vi "Init Open Error Logs Folder Button.vi"(8 "Error In":errorcluster, 10 "Error_Log_Setting":T1, 11 "Open Error Logs Folder Button Reference":refnum<vi>) -> (0 "Error Out":errorcluster)   [LabVIEW 2023, in "Error Manager.lvlib"]
doc: "Blank VI with error handling."
uses:
  Error Manager.lvlib
  Settings/Error_Log_Setting (enum).ctl
  Settings/Settings.lvclass
panel:
  # "Input\nInputs to the VI"
  # "Development\nControls or indicators that are useful for development or testing, but which are not outputs of the VI."
  # "Output\nOutputs of the VI"
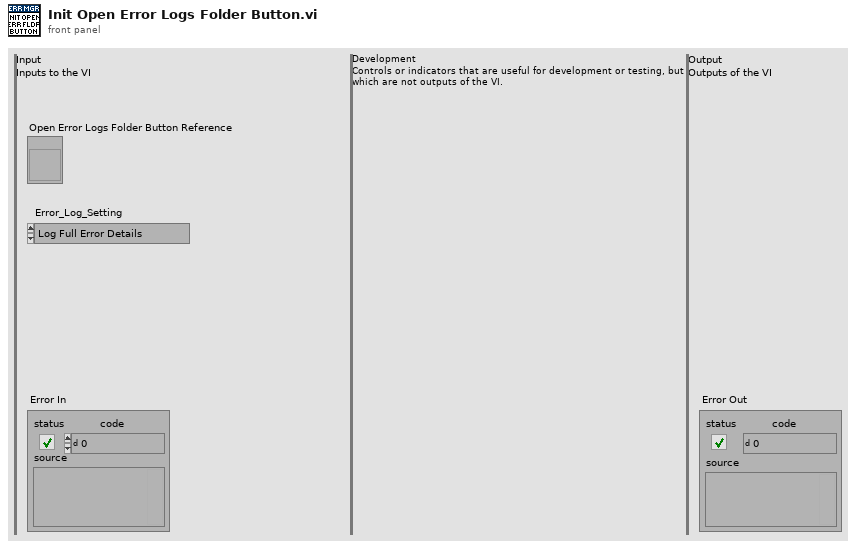
[diagram p1: front panel]
types:
  T1 = typedef "Error Manager.lvlib/Settings.lvclass/Error_Log_Setting (enum).ctl" = enum16{"Log Full Error Details", "Log Error Codes Only", "Do Not Log"}
  T2 = enum8{"Enabled", "Disabled", "Disabled and Grayed Out"}
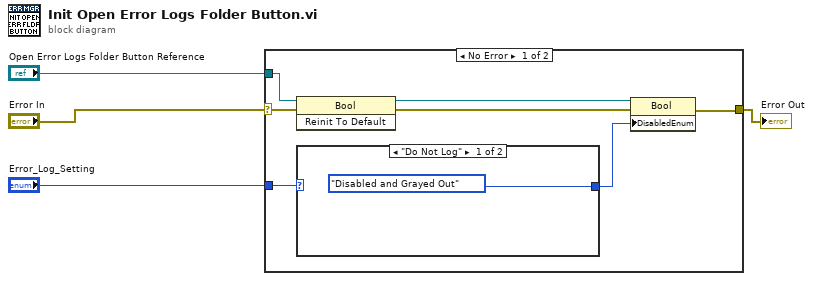
[diagram p0: block diagram]
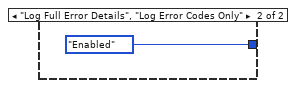
[diagram p2: hidden frame]
diagram:
  n1 = case shown="No Error" "Error In" {
    selector: "Error In" -> [w11 w14]
    tunnel: [w10 w14] -> w3
    tunnel: "Open Error Logs Folder Button Reference" -> [w6 _]
    tunnel: "Error_Log_Setting" -> [w9 _]
    frame No Error {
      n2 = invoke class="Bool" method="Reinit To Default"(reference=w6, error in=w11) -> (reference out=w5:refnum<vi>, error out=w7:errorcluster)  [unwired: 1 in, 1 out]
      n3 = case shown="\"Do Not Log\"" w9 {
        tunnel: [T2."Disabled and Grayed Out" ("Disabled") T2."Enabled" ("Disabled")] -> w8
        frame "Do Not Log" {
        }
        frame "Log Full Error Details", "Log Error Codes Only" {
        }
      }
      n4 = property class="Bool"(reference=w5, error in=w7, "DisabledEnum"=w8) -> (error out=w10:errorcluster)  [unwired: 1 out]
    }
    frame Error {
    }
  }
  "Error Out" <- w3
